vi "Receiver_Example - 2 Channel - Experiment_2.vi"() -> ()   [LabVIEW 2022 SP3]
panel:
  out "iterationsIM  2":dbl
  out "iterationsIM":dbl
  out "High-Power Image 2":T1(plugin-control)
  out "High-Power Decoded message - CH0":string
  out "High-Power BER - CH0":dbl(graph)
  in  "High-Power Window Size - CH0":dbl=15.0 format="%#_6p"
  out "High-Power BER - CH1":dbl(graph)
  in  "High-Power Window Size - CH1":dbl=15.0 format="%#_6p"
  in  "Low-Power Window Size - CH0":dbl=15.0 format="%#_6p"
  out "Low-Power BER - CH0":dbl(graph)
  out "Constellation Map":cluster{"Constellation":cdb[]}[](graph)
  in  "Tab Control":enum32{"USRP Parameters", "Rx Info", "BER"}(tab)
  in  "USRP ControledParameters":T2={"Active Antenna"="RX2", "Gain (dB)"=10.0, "Carrier Frequency"=2400000000.0, "IQ Rate"=2000000.0, "Active channels"="0,1"} {"IQ Rate" format="%#_6p"; "Carrier Frequency" format="%#_6p"; "Gain (dB)" format="%#_6f"}
  in  "Device selection":refnum<k15>="RIO0"
  in  "Trigger level":dbl=0.005 format="%f"
  out "CH0":T3
  out "CH1":T3
  out "SIG valid? - CH1":bool
  out "SIG valid? - CH0":bool
  out "Frequency offset - CH1":dbl
  out "Frequency offset - CH0":dbl
  out "Coerced Parameters":T4={"IQ Rate"=100000.0, "Carrier  Freq."=100000.0, "Gain"=0.0} {"Gain" format="%#_6f"; "Carrier  Freq." format="%#_6p"; "IQ Rate" format="%#_6p"}
  out "Error out":errorcluster
  in  "Expected message LP - CH0":string="Non Critical Data\nNon Critical Data\nNon Critical Data\nNon Critical Data\nNon Critical Data"
  in  "Expected message - CH1":string="Critical Dataaaaa\nCritical Dataaaaa\nCritical Dataaaaa\nCritical Dataaaaa\nCritical Dataaaaa"
  out "Expected message LP Detected CH0":string="Non Critical Data\nNon Critical Data\nNon Critical Data\nNon Critical Data\nNon Critical Data"
  out "Expected message HP Detected CH1":string="Non Critical Data\nNon Critical Data\nNon Critical Data\nNon Critical Data\nNon Critical Data"
  in  "Boolean":bool
  in  "Boolean 3":bool
  out "Expected message HP Detected CH0":string="Non Critical Data\nNon Critical Data\nNon Critical Data\nNon Critical Data\nNon Critical Data"
  in  "Expected message HP - CH0":string="Critical Dataaaaa\nCritical Dataaaaa\nCritical Dataaaaa\nCritical Dataaaaa\nCritical Dataaaaa"
  in  "Boolean 2":bool
  out "Inst. BER HP - CH0":dbl format="%#_4g"
  out "Acc. BER HP - CH0":dbl format="%#_4g"
  out "Acum. Err HP - CH0":dbl
  out "No. Bits HP - CH0":dbl
  out "Acc. BER LP - CH0":dbl format="%#_4g"
  out "Inst. BER - CH1":dbl format="%#_4g"
  out "Inst. BER LP - CH0":dbl format="%#_4g"
  out "No. Bits - CH1":dbl
  out "No. Bits LP - CH0":dbl
  out "Acum. Err - CH1":dbl
  out "Acum. Err LP - CH0":dbl
  in  "Record BER":bool
  in  "Refresh Button":bool
  out "Acc. BER - CH1":dbl format="%#_4g"
  in  "error in (no error)":errorcluster
  out "Decoded message - CH1":string
  out "Low-Power Decoded message - CH0":string
  # "OFDM Superposition Coded Receiver"
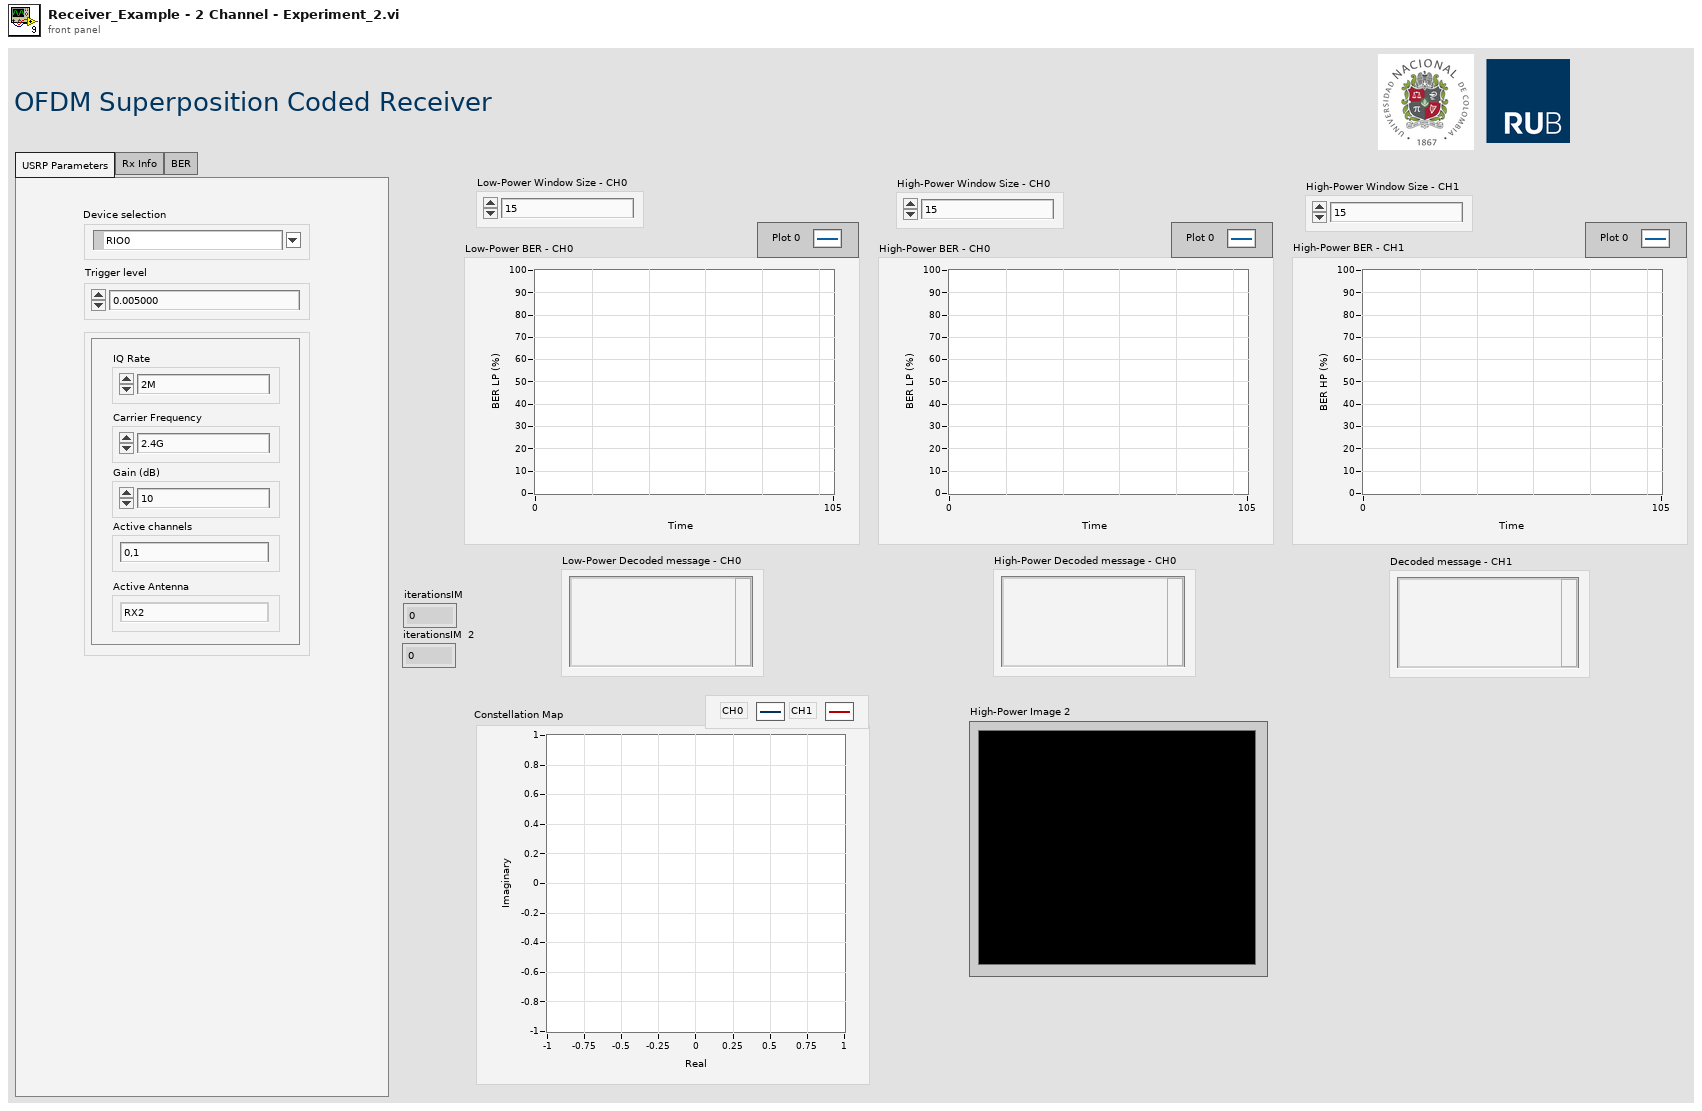
[diagram p1: front panel]
types:
  T1 = typedef "IMAQ Image.ctl" = refnum<image>
  T2 = cluster{"Active Antenna":string, "Gain (dB)":dbl, "Carrier Frequency":dbl, "IQ Rate":dbl, "Active channels":string}
  T3 = cluster{"Modulation type":enum16{"QPSK(4QAM)", "64QAM", "16QAM", "BPSK"}, "BCC rate (k/n)":enum16{"1/2", "2/3", "3/4"}}
  T4 = cluster{"IQ Rate":dbl, "Carrier  Freq.":dbl, "Gain":dbl}
  T5 = cluster{"coerced IQ rate":dbl, "coerced carrier frequency":dbl, "coerced gain":dbl}
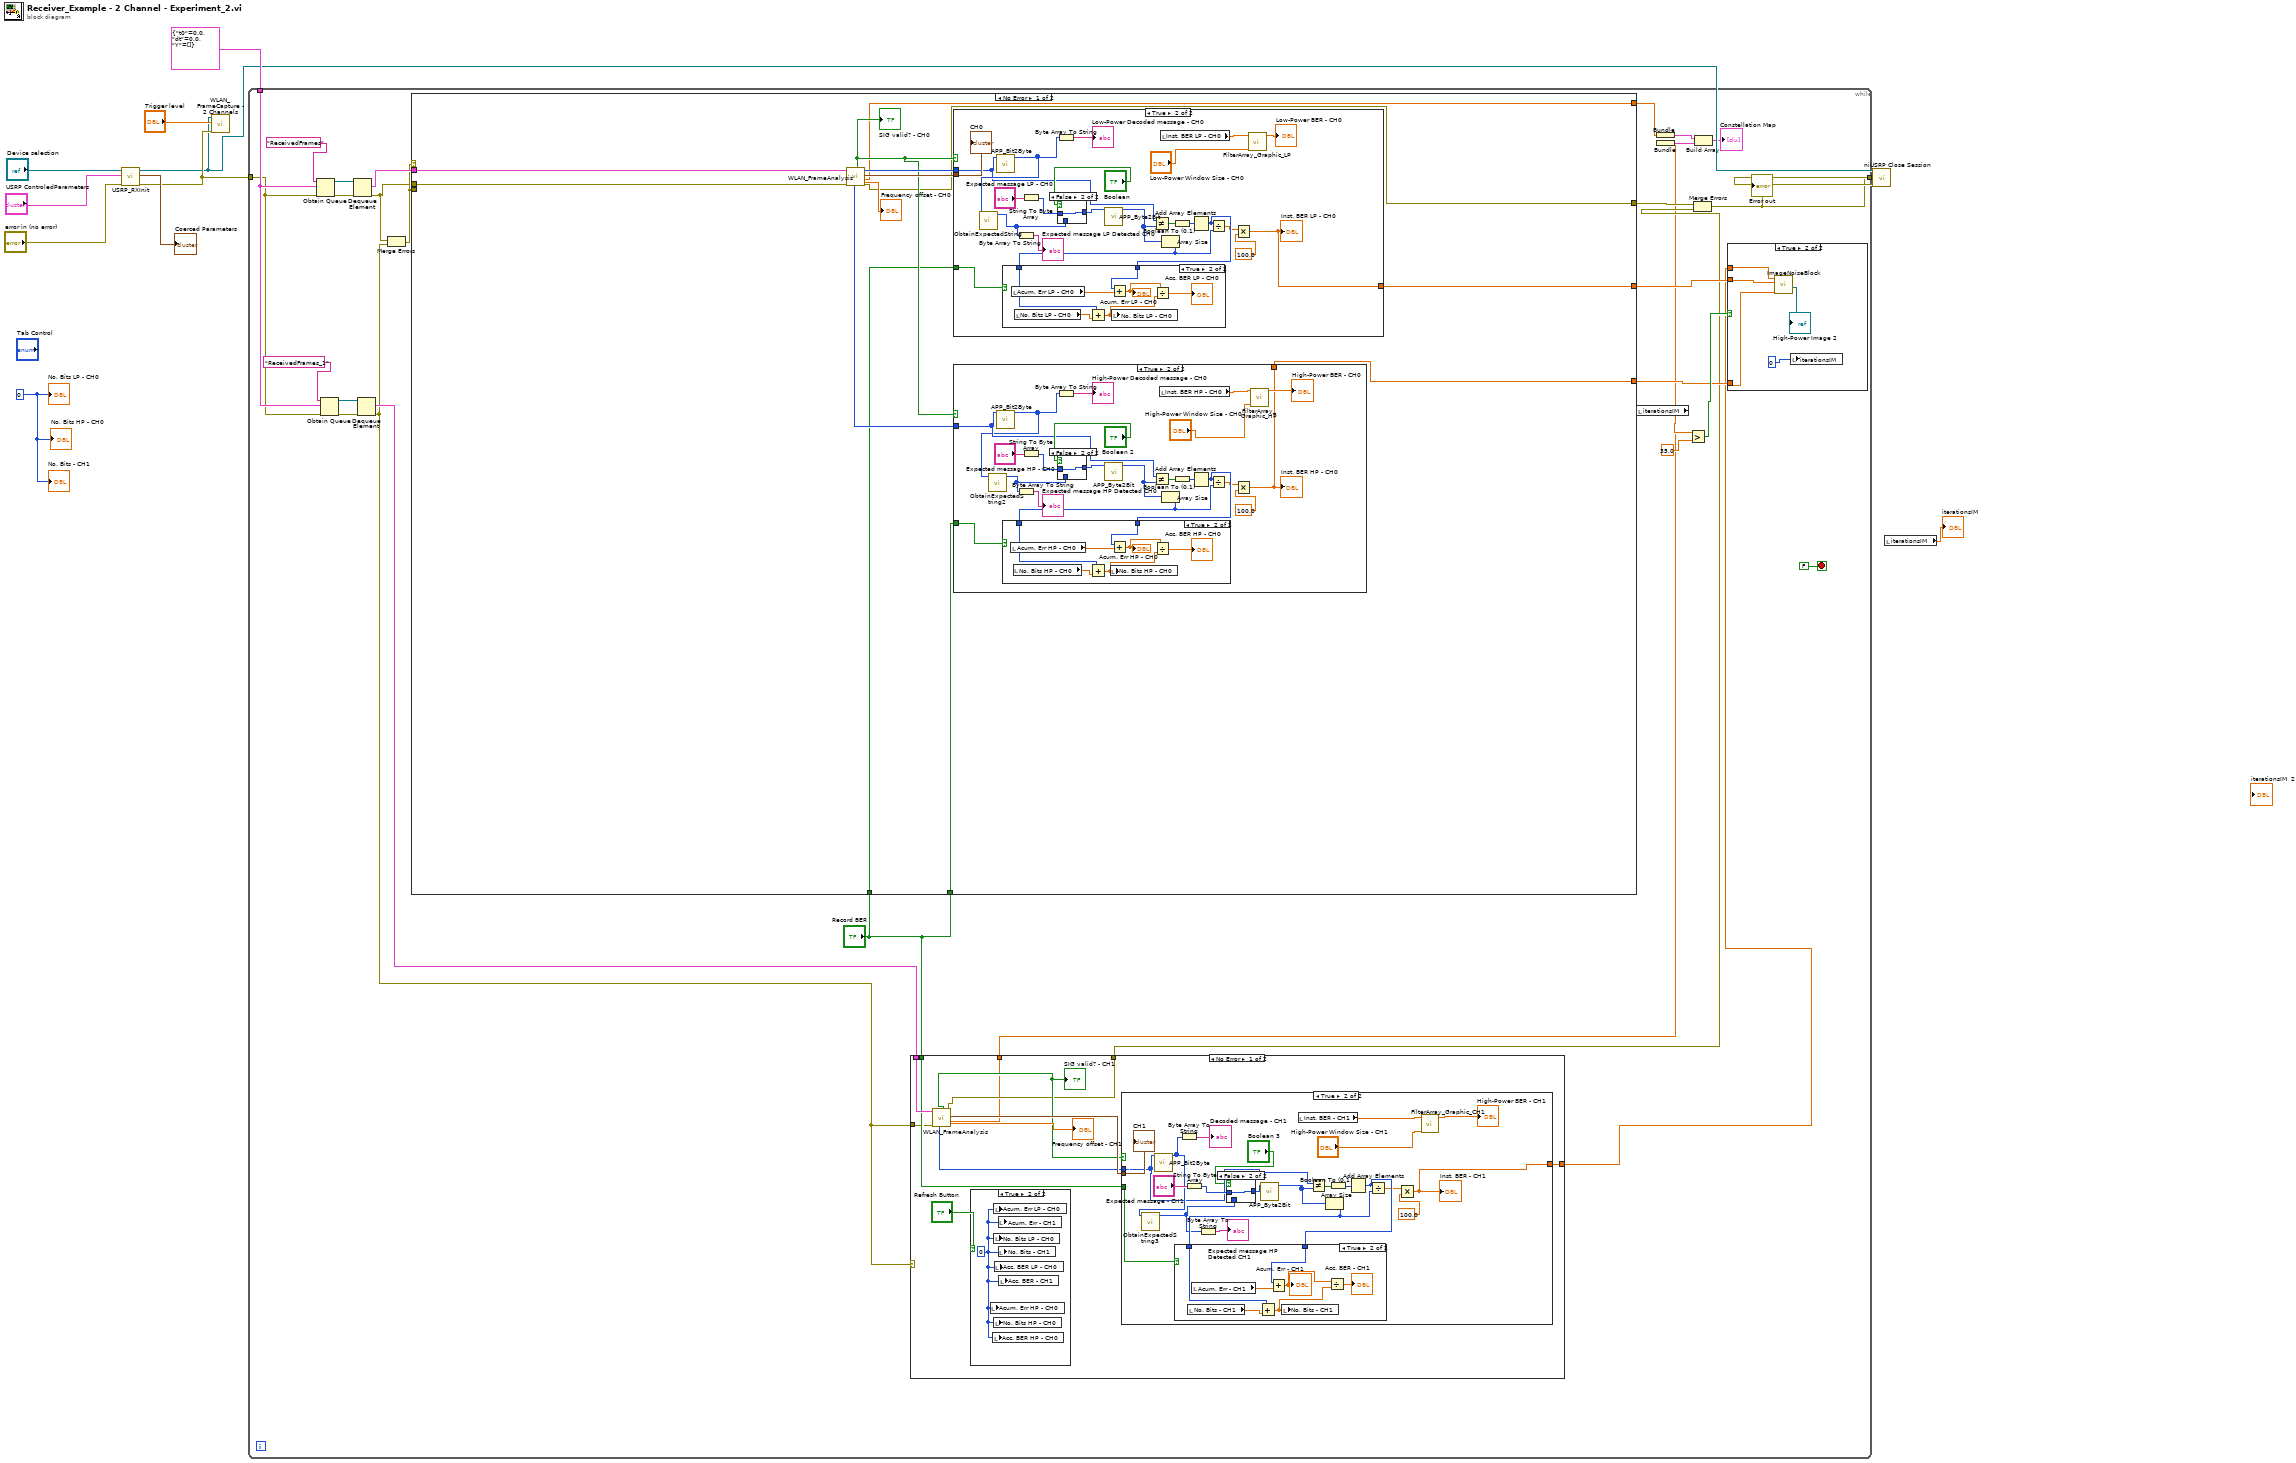
[diagram p0: block diagram]
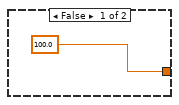
[diagram p3: hidden frame]
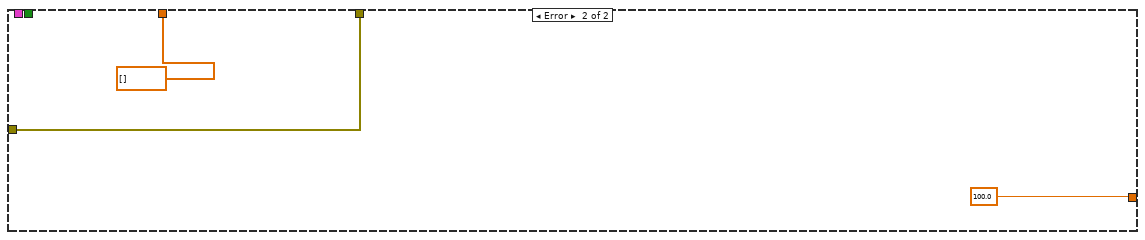
[diagram p6: hidden frame]
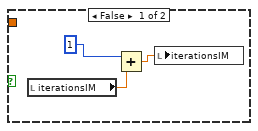
[diagram p7: hidden frame]
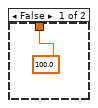
[diagram p8: hidden frame]
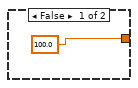
[diagram p11: hidden frame]
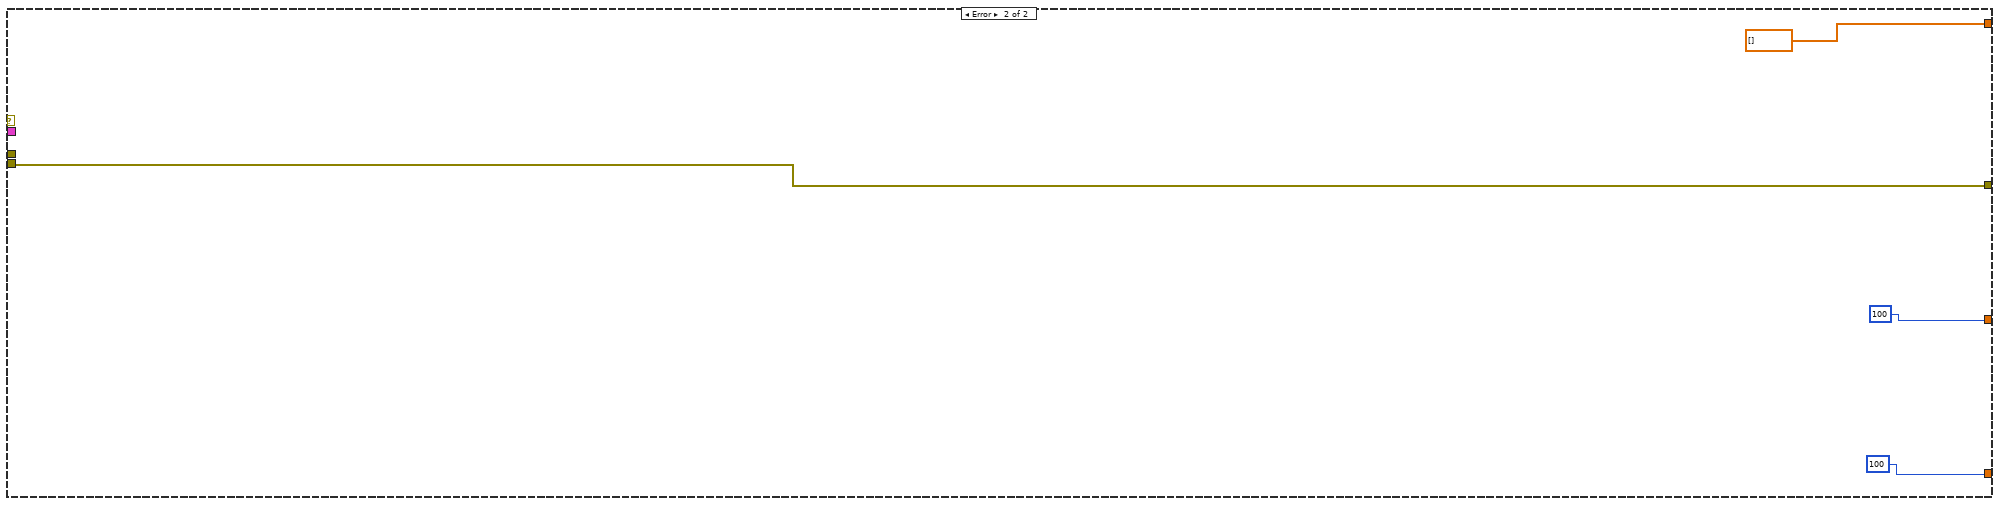
[diagram p14: hidden frame]
diagram:
  w2 = 0
  n1 = call "USRP_RXInit.vi"("device names"="Device selection", "USRP ControledParameters"="USRP ControledParameters", "error in (no error)"="error in (no error)") -> ("session handle out"=w5:refnum<k15>, "USRP CoercedParamters"=→"Coerced Parameters":T5, "error out"=w9:errorcluster)  [unwired: 5 in]
  n2 = call "WLAN_FrameCapture - 2 Channels.vi"("error in (no error)"=w9, "Trigger level"="Trigger level", "session handle"=w5) -> ()  [unwired: 8 in]
  n3 = while {
    tunnel: w9 -> [w32]
    tunnel: cluster{"t0":dbl, "dt":dbl, "Y":cdb[]} {"t0"=0.0, "dt"=0.0, "Y"=[]} ("data") -> [w33]
    tunnel: [w15] -> w6
    stop <- FALSE stop-if-true
    n4 = Obtain Queue(name (unnamed)="ReceivedFrames", element data type=w33, error in (no error)=w32) -> (queue out=w40:refnum<queue>, error out=w38:errorcluster)  [unwired: 2 in, 1 out]
    n5 = Obtain Queue(name (unnamed)="ReceivedFrames_1", element data type=w33, error in (no error)=w32) -> (queue out=w36:refnum<queue>, error out=w35:errorcluster)  [unwired: 2 in, 1 out]
    n6 = Dequeue Element(queue=w40, error in (no error)=w38) -> (element=w39:cluster{"t0":dbl, "dt":dbl, "Y":cdb[]}, error out=w29:errorcluster)  [unwired: 1 in, 2 out]
    n7 = Dequeue Element(queue=w36, error in (no error)=w35) -> (element=w18:cluster{"t0":dbl, "dt":dbl, "Y":cdb[]}, error out=w13:errorcluster)  [unwired: 1 in, 2 out]
    n8 = Merge Errors(w29, w13) -> (w30:errorcluster)
    n9 = case shown="No Error" w30 {
      tunnel: w39 -> [w105 _]
      tunnel: w30 -> [_ w173]
      tunnel: w29 -> [w102 _]
      tunnel: [w101 100] -> w25
      tunnel: [w100 100] -> w24
      tunnel: [w99 dbl[] []] -> w20
      tunnel: [w98 w173] -> w17
      tunnel: "Record BER" -> [w97 _]
      tunnel: "Record BER" -> [w96 _]
      frame No Error {
        n10 = call "WLAN_FrameAnalysis.vi"("error in (no error)"=w102, "input cluster"=w105) -> ("error out"=w98:errorcluster, "Constellation"=w99:cdb[], "Modulation parameter"=w106:T3, "output bits"=w107:i8[], "Frequency offset"=→"Frequency offset - CH0":dbl, "SIG valid?"=w103:bool, "outputbitsHP"=w104:i8[])  [unwired: 3 in]
        "SIG valid? - CH0" <- w103
        n11 = case shown="True" w103 {
          tunnel: w107 -> [_ w142]
          tunnel: w106 -> [_ w161]
          tunnel: w96 -> [_ w157]
          tunnel: [100.0 w141] -> w101
          frame False {
          }
          frame True {
            n12 = call "APP_Bit2Byte.vi"("input bit stream"=w142) -> ("output byte stream"=w146:u8[])  [unwired: 10 in]
            n13 = call "ObtainExpectedString.vi"("Array"=w146) -> ("detectedMessage"=w143:i8[])  [unwired: 9 in]
            n14 = Byte Array To String(unsigned byte array=w143) -> (string=→"Expected message LP Detected CH0":string)
            n15 = String To Byte Array(string="Expected message LP - CH0") -> (unsigned byte array=w147:u8[])
            n16 = Byte Array To String(unsigned byte array=w146) -> (string=→"Low-Power Decoded message - CH0":string)
            n17 = case shown="False" "Boolean" {
              tunnel: [w163 w164] -> w149
              tunnel: w147 -> [_ w164]
              tunnel: w143 -> [w163 _]
              frame True {
              }
              frame False {
              }
            }
            n18 = call "APP_Byte2Bit.vi"("input byte stream"=w149) -> ("output bit stream"=w148:i8[])  [unwired: 10 in]
            n19 = Not Equal?(x=w142, y=w148) -> (x != y?=w159:bool[])
            n20 = local read "Inst. BER LP - CH0"() -> (w152:dbl)
            n21 = Array Size(array=w148) -> (size(s)=w156:i32)
            n22 = Boolean To (0,1)(Boolean=w159) -> (0, 1=w160:i16[])
            n23 = Add Array Elements(numeric array=w160) -> (sum=w155:i16)
            n24 = case shown="True" w157 {
              tunnel: w156 -> [_ w170]
              tunnel: w155 -> [_ w168]
              frame False {
              }
              frame True {
                n25 = local read "Acum. Err LP - CH0"() -> (w169:dbl)
                n26 = local read "No. Bits LP - CH0"() -> (w171:dbl)
                n27 = Add(x=w170, y=w171) -> (x+y=w167:dbl)
                n28 = Add(x=w168, y=w169) -> (x+y=w166:dbl)
                "Acum. Err LP - CH0" <- w166
                n29 = local write "No. Bits LP - CH0"(w167) -> ()
                n30 = Divide(x=w166, y=w167) -> (x/y=→"Acc. BER LP - CH0":dbl)
              }
            }
            n31 = Divide(x=w155, y=w156) -> (x/y=w151:dbl)
            n32 = Multiply(x=w151, y=100.0) -> (x*y=w141:dbl)
            "Inst. BER LP - CH0" <- w141
            n33 = call "FilterArray_Graphic_LP.vi"("Window Size"="Low-Power Window Size - CH0", "Instantaneous BER"=w152) -> ("Graph Instantaneous BER"=→"Low-Power BER - CH0":dbl)  [unwired: 4 in, 1 out]
            "CH0" <- w161
          }
        }
        n34 = case shown="True" w103 {
          tunnel: w104 -> [_ w116]
          tunnel: w97 -> [_ w126]
          tunnel: [100.0 w110] -> w100
          frame False {
          }
          frame True {
            n35 = call "APP_Bit2Byte.vi"("input bit stream"=w116) -> ("output byte stream"=w113:u8[])  [unwired: 10 in]
            n36 = call "ObtainExpectedString2.vi"("Array"=w113) -> ("detectedMessage"=w112:i8[])  [unwired: 9 in]
            n37 = Byte Array To String(unsigned byte array=w112) -> (string=→"Expected message HP Detected CH0":string)
            n38 = String To Byte Array(string="Expected message HP - CH0") -> (unsigned byte array=w119:u8[])
            n39 = Byte Array To String(unsigned byte array=w113) -> (string=→"High-Power Decoded message - CH0":string)
            n40 = case shown="False" "Boolean 2" {
              tunnel: [w131 w132] -> w121
              tunnel: w119 -> [_ w132]
              tunnel: w112 -> [w131 _]
              frame True {
              }
              frame False {
              }
            }
            n41 = call "APP_Byte2Bit.vi"("input byte stream"=w121) -> ("output bit stream"=w120:i8[])  [unwired: 10 in]
            n42 = Not Equal?(x=w116, y=w120) -> (x != y?=w128:bool[])
            n43 = local read "Inst. BER HP - CH0"() -> (w111:dbl)
            n44 = Array Size(array=w120) -> (size(s)=w125:i32)
            n45 = Boolean To (0,1)(Boolean=w128) -> (0, 1=w129:i16[])
            n46 = Add Array Elements(numeric array=w129) -> (sum=w124:i16)
            n47 = case shown="True" w126 {
              tunnel: w125 -> [_ w138]
              tunnel: w124 -> [_ w136]
              frame False {
              }
              frame True {
                n48 = local read "Acum. Err HP - CH0"() -> (w137:dbl)
                n49 = local read "No. Bits HP - CH0"() -> (w139:dbl)
                n50 = Add(x=w138, y=w139) -> (x+y=w135:dbl)
                n51 = local write "No. Bits HP - CH0"(w135) -> ()
                n52 = Add(x=w136, y=w137) -> (x+y=w134:dbl)
                "Acum. Err HP - CH0" <- w134
                n53 = Divide(x=w134, y=w135) -> (x/y=→"Acc. BER HP - CH0":dbl)
              }
            }
            n54 = Divide(x=w124, y=w125) -> (x/y=w123:dbl)
            n55 = Multiply(x=w123, y=100.0) -> (x*y=w110:dbl)
            "Inst. BER HP - CH0" <- w110
            n56 = call "FilterArray_Graphic_HP.vi"("Window Size"="High-Power Window Size - CH0", "Instantaneous BER"=w111) -> ("Graph Instantaneous BER"=→"High-Power BER - CH0":dbl)  [unwired: 4 in, 1 out]
          }
        }
      }
      frame Error {
      }
    }
    n57 = case shown="No Error" w13 {
      tunnel: [w47 100.0] -> w19
      tunnel: w18 -> [w46 _]
      tunnel: "Record BER" -> [w44 _]
      tunnel: [w43 w86] -> w16
      tunnel: [w42 dbl[] []] -> w14
      tunnel: w13 -> [w41 w86]
      frame No Error {
        n58 = call "WLAN_FrameAnalysis.vi"("error in (no error)"=w41, "input cluster"=w46) -> ("error out"=w43:errorcluster, "Constellation"=w42:cdb[], "Modulation parameter"=w50:T3, "Frequency offset"=→"Frequency offset - CH1":dbl, "SIG valid?"=w45:bool, "outputbitsHP"=w48:i8[])  [unwired: 3 in, 1 out]
        "SIG valid? - CH1" <- w45
        n59 = case shown="True" "Refresh Button" {
          frame False {
          }
          frame True {
            w52 = 0
            n60 = local write "Acum. Err HP - CH0"(w52) -> ()
            n61 = local write "Acc. BER HP - CH0"(w52) -> ()
            n62 = local write "Acum. Err LP - CH0"(w52) -> ()
            n63 = local write "No. Bits LP - CH0"(w52) -> ()
            n64 = local write "No. Bits HP - CH0"(w52) -> ()
            n65 = local write "Acc. BER LP - CH0"(w52) -> ()
            n66 = local write "Acum. Err - CH1"(w52) -> ()
            n67 = local write "No. Bits - CH1"(w52) -> ()
            n68 = local write "Acc. BER - CH1"(w52) -> ()
          }
        }
        n69 = case shown="True" w45 {
          tunnel: w48 -> [_ w60]
          tunnel: w50 -> [_ w75]
          tunnel: [100.0 w55] -> w47
          tunnel: w44 -> [_ w54]
          frame False {
          }
          frame True {
            n70 = call "APP_Bit2Byte.vi"("input bit stream"=w60) -> ("output byte stream"=w63:u8[])  [unwired: 10 in]
            n71 = call "ObtainExpectedString3.vi"("Array"=w63) -> ("detectedMessage"=w62:i8[])  [unwired: 9 in]
            n72 = Byte Array To String(unsigned byte array=w63) -> (string=→"Decoded message - CH1":string)
            n73 = String To Byte Array(string="Expected message - CH1") -> (unsigned byte array=w64:u8[])
            n74 = Byte Array To String(unsigned byte array=w62) -> (string=→"Expected message HP Detected CH1":string)
            n75 = case shown="False" "Boolean 3" {
              tunnel: [w76 w77] -> w66
              tunnel: w64 -> [_ w77]
              tunnel: w62 -> [w76 _]
              frame True {
              }
              frame False {
              }
            }
            n76 = call "APP_Byte2Bit.vi"("input byte stream"=w66) -> ("output bit stream"=w65:i8[])  [unwired: 10 in]
            n77 = local read "Inst. BER - CH1"() -> (w58:dbl)
            n78 = Not Equal?(x=w60, y=w65) -> (x != y?=w72:bool[])
            n79 = Array Size(array=w65) -> (size(s)=w70:i32)
            n80 = Boolean To (0,1)(Boolean=w72) -> (0, 1=w73:i16[])
            n81 = Add Array Elements(numeric array=w73) -> (sum=w69:i16)
            n82 = case shown="True" w54 {
              tunnel: w70 -> [_ w83]
              tunnel: w69 -> [_ w81]
              frame False {
              }
              frame True {
                n83 = local read "No. Bits - CH1"() -> (w84:dbl)
                n84 = local read "Acum. Err - CH1"() -> (w82:dbl)
                n85 = Add(x=w83, y=w84) -> (x+y=w80:dbl)
                n86 = Add(x=w81, y=w82) -> (x+y=w79:dbl)
                "Acum. Err - CH1" <- w79
                n87 = local write "No. Bits - CH1"(w80) -> ()
                n88 = Divide(x=w79, y=w80) -> (x/y=→"Acc. BER - CH1":dbl)
              }
            }
            n89 = Divide(x=w69, y=w70) -> (x/y=w67:dbl)
            n90 = Multiply(x=w67, y=100.0) -> (x*y=w55:dbl)
            "Inst. BER - CH1" <- w55
            n91 = call "FilterArray_Graphic_CH1.vi"("Window Size"="High-Power Window Size - CH1", "Instantaneous BER"=w58) -> ("Graph Instantaneous BER"=→"High-Power BER - CH1":dbl)  [unwired: 4 in, 1 out]
            "CH1" <- w75
          }
        }
      }
      frame Error {
      }
    }
    n92 = local read "iterationsIM"() -> (w28:dbl)
    n93 = Bundle("Constellation"=w20) -> (w23:cluster{"Constellation":cdb[]})  [unwired: 1 in]
    n94 = Bundle("Constellation"=w14) -> (w22:cluster{"Constellation":cdb[]})  [unwired: 1 in]
    n95 = Greater?(x=w28, y=35.0) -> (0:w27:bool)
    n96 = Merge Errors(w17, w16) -> (w15:errorcluster)
    "Error out" <- w15
    n97 = Build Array(w23, w22) -> (→"Constellation Map":cluster{"Constellation":cdb[]}[])
    n98 = case shown="True" w27 {
      tunnel: w19 -> [_ w95]
      tunnel: w25 -> [_ w94]
      tunnel: w24 -> [_ w93]
      frame False {
        n99 = local read "iterationsIM"() -> (w90:dbl)
        n100 = Add(x=1, y=w90) -> (x+y=w89:dbl)
        n101 = local write "iterationsIM"(w89) -> ()
      }
      frame True {
        n102 = call "ImageNoiseBlock.vi"("BERCOMP"=w95, "BERLP"=w94, "BERHP"=w93) -> ("High-Power Image"=→"High-Power Image 2":T1)  [unwired: 7 in]
        n103 = local write "iterationsIM"(0) -> ()
      }
    }
  }
  n104 = call <instrlib>:"niUSRP Close Session.vi"("session handle"=w5, "error in (no error)"=w6) -> ()  [unwired: 13 in, 1 out]
  n105 = local read "iterationsIM"() -> (→"iterationsIM":dbl)
  "No. Bits LP - CH0" <- w2
  "No. Bits - CH1" <- w2
  "No. Bits HP - CH0" <- w2
